vi "Clock Frequency generator hilbert.vi"(6 "Sweep Speed":dbl=20000.0 format="%#_13g", 8 "Error In":errorcluster, 9 "Acquisition speed (S/s)":i32=180000000, 10 "k-space signal in":u16[](array[numeric])=array[5000 elements], 11 "number of frequency updates":i32=4385) -> (0 "Error Out":errorcluster, 2 "frequency\nsteps":i32)   [LabVIEW 2014]
uses:
  <vilib>/Analysis/polynomials.llb/nth Derivative of Polynomial (DBL).vi
  <vilib>/Analysis/polynomials.llb/Scalar Polynomial Evaluation (DBL).vi
  <vilib>/Analysis/NI_AALPro.lvlib
panel:
  out "Frequency output 2":cluster{dbl[], dbl[]}[](graph)
  out "x*y":dbl[](array[numeric])
  out "Update time interval (ns)":dbl=10.0
  out "Frequency output":dbl[](graph)
  out "analytic phase":dbl[][](graph)
  in  "End of clock":i32=6300
  out "original signal":dbl[](graph)
  # "4385 updates is the maximum number for the clock of\nthe output card which updates every 11.4 ns"
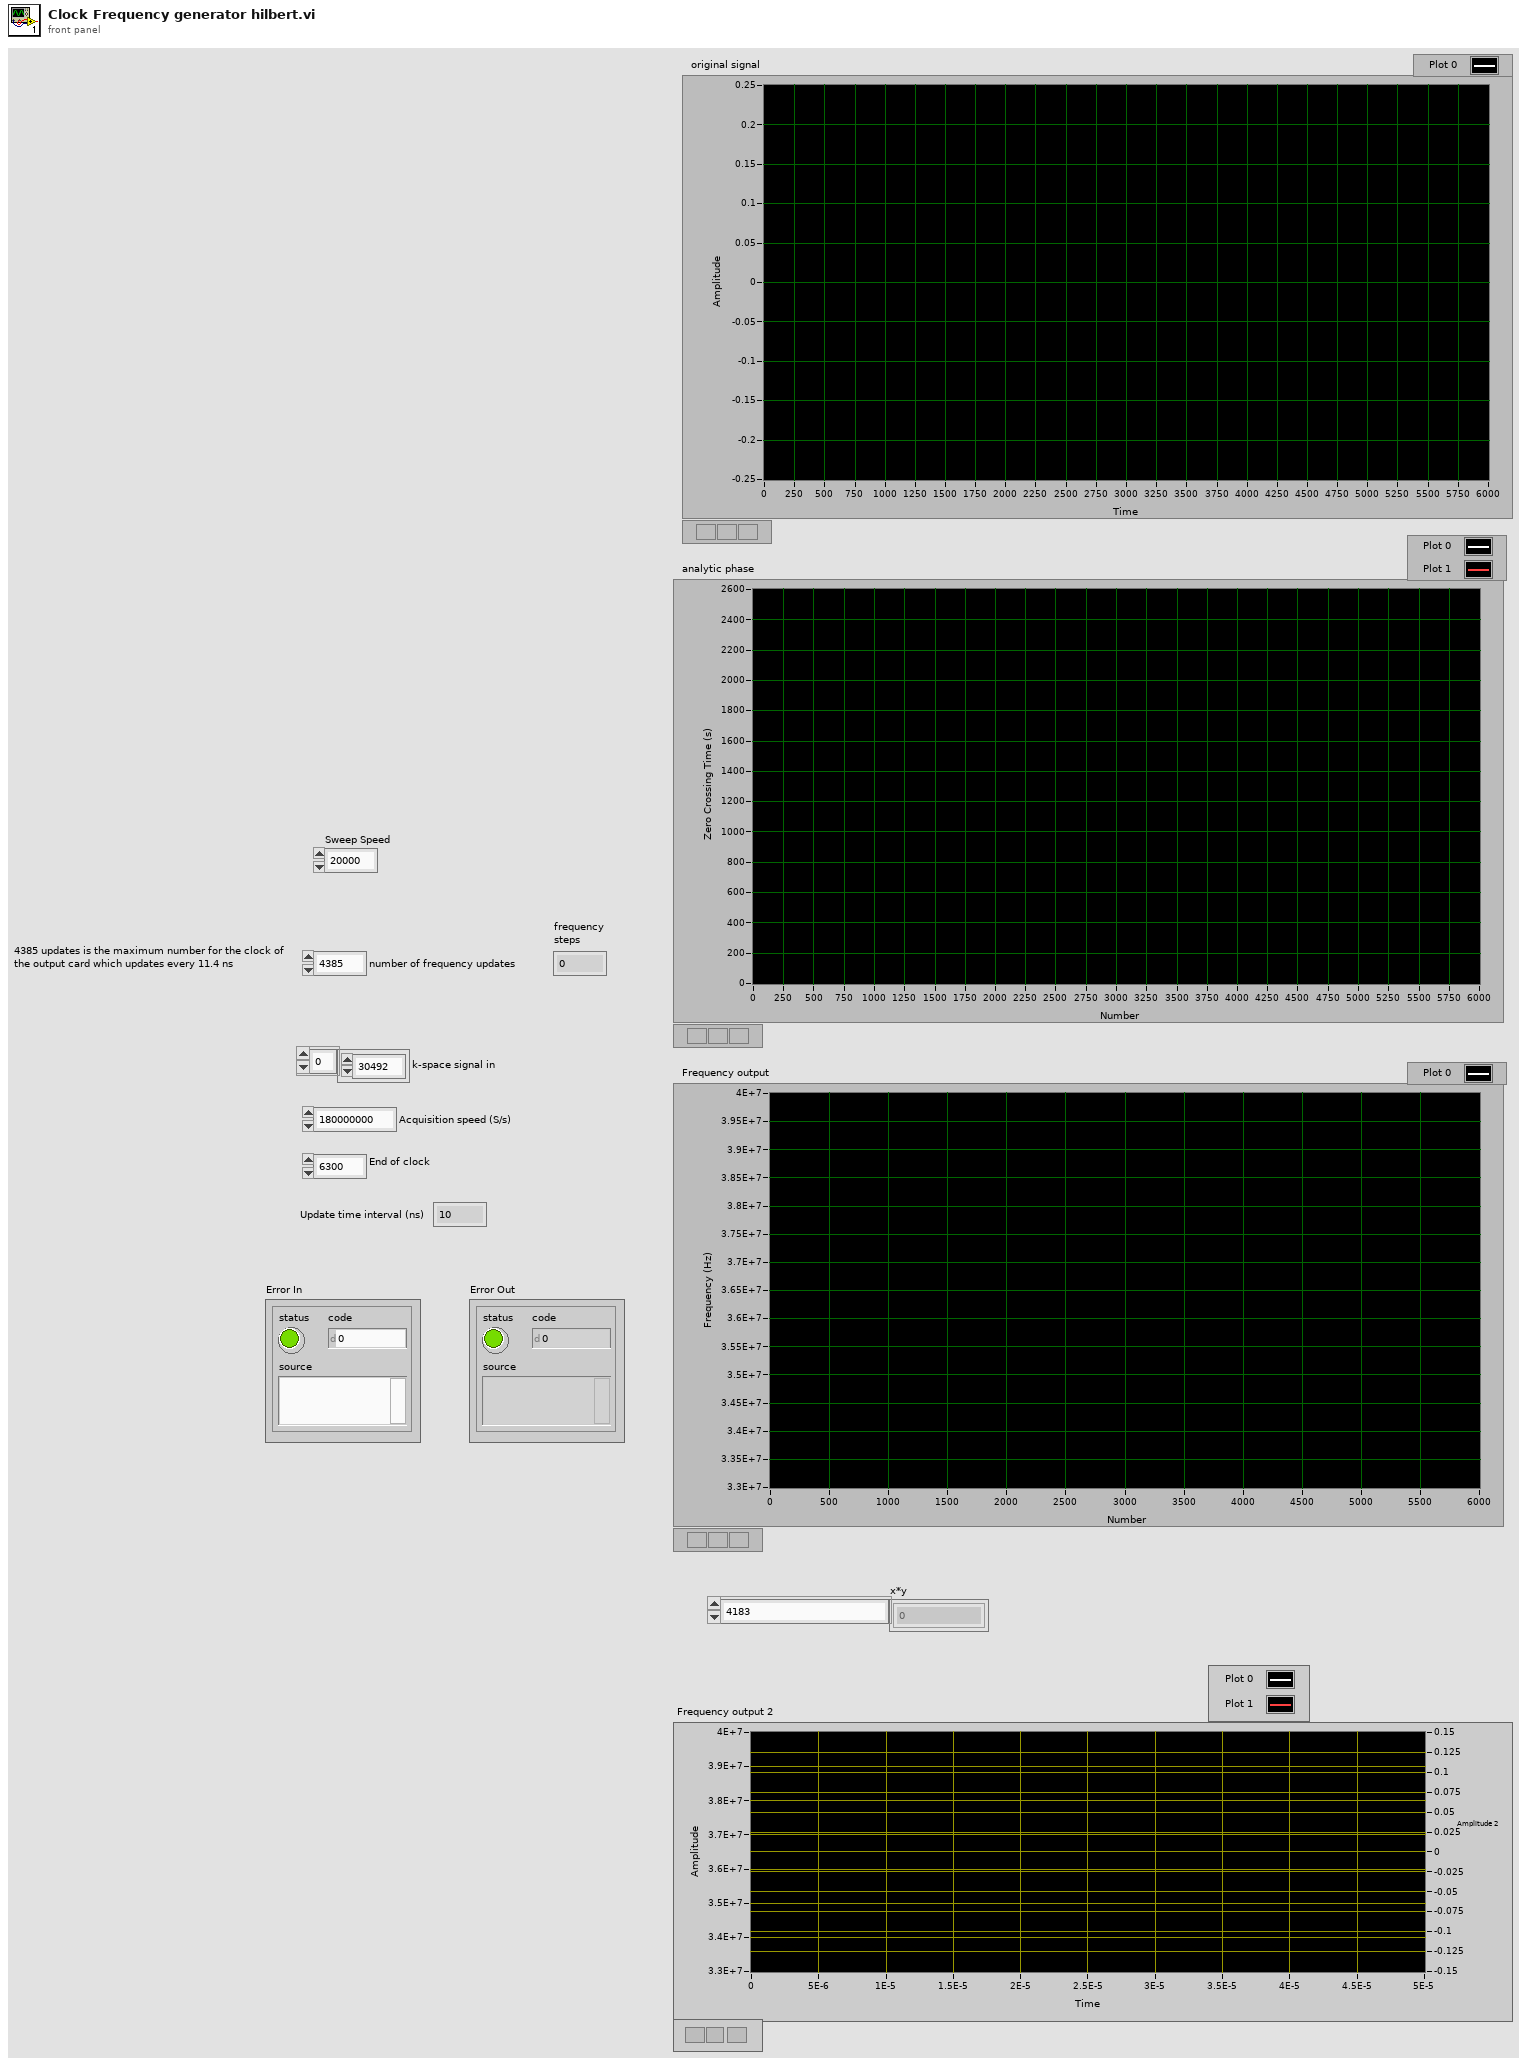
[diagram p1: front panel]
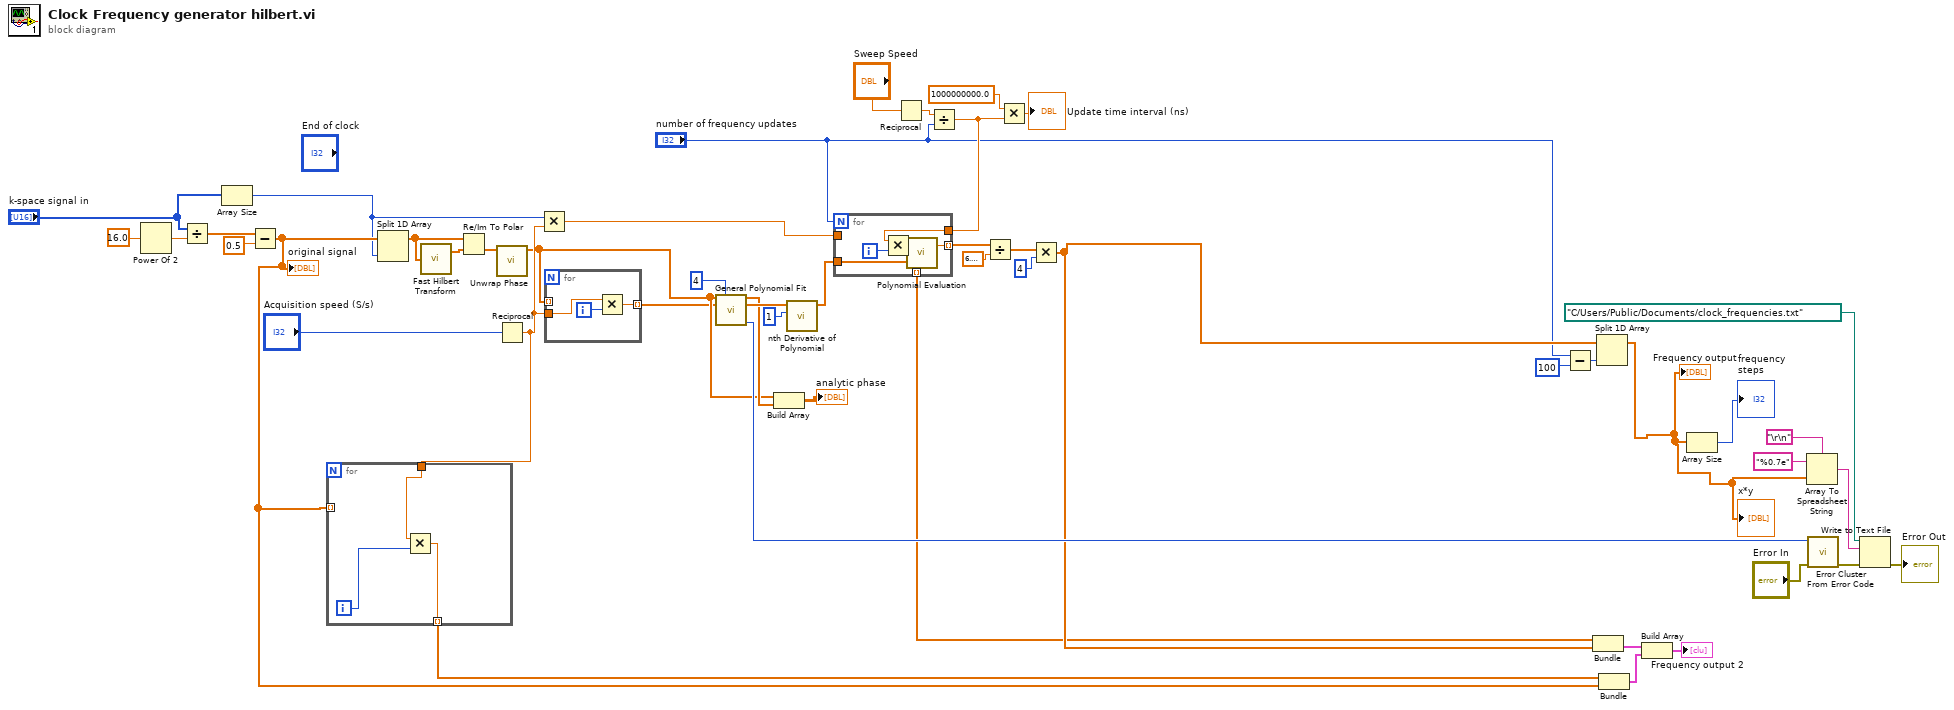
[diagram p0: block diagram]
diagram:
  n1 = Power Of 2(x=16.0) -> (2^x=w49:dbl)
  n2 = Divide(x="k-space signal in", y=w49) -> (x/y=w47:dbl[])
  n3 = Array Size(array="k-space signal in") -> (size(s)=w1:i32)
  n4 = Subtract(x=w47, y=0.5) -> (x-y=w12:dbl[])
  "original signal" <- w12
  n5 = Split 1D Array(array=w12, index=w1) -> (first subarray=w23:dbl[])  [unwired: 1 out]
  n6 = call <vilib>:"Fast Hilbert Transform.vi"("X"=w23) -> ("Hilbert{X}"=w26:dbl[])  [unwired: 1 out]
  n7 = Re/Im To Polar(2:w26, 3:w23) -> (0:w25:dbl[])  [unwired: 1 out]
  n8 = call <vilib>:"Unwrap Phase.vi"("Phase"=w25) -> ("Unwrapped Phase"=w8:dbl[])  [unwired: 9 in, 1 out]
  n9 = Reciprocal(x="Acquisition speed (S/s)") -> (1/x=w11:dbl)
  n10 = for {
    tunnel: w12 -> [_] mode=indexing
    tunnel: w11 -> [w52]
    tunnel: [w50] -> w9 mode=indexing
    i -> [w51]
    n11 = Multiply(x=w52, y=w51) -> (x*y=w50:dbl)
  }
  n12 = Multiply(x=w1, y=w11) -> (x*y=w22:dbl)
  n13 = for {
    tunnel: w8 -> [_] mode=indexing
    tunnel: [w54] -> w7 mode=indexing
    tunnel: w11 -> [w53]
    i -> [w55]
    n14 = Multiply(x=w53, y=w55) -> (x*y=w54:dbl)
  }
  n15 = call <vilib>:"General Polynomial Fit.vi"("Y"=w8, "polynomial order"=4, "X"=w7) -> ("Best Polynomial Fit"=w33:dbl[], "Polynomial Coefficients"=w36:dbl[], "error"=w30:i32)  [unwired: 9 in, 1 out]
  n16 = Build Array(w8, w33) -> (→"analytic phase":dbl[][])
  n17 = call-poly <vilib>:"nth Derivative of Polynomial.vi"("order"=1, "P(x)"=w36) -> ("Nth Derivative of P(x)"=w31:dbl[])  [unwired: 8 in, 1 out]
  n18 = Reciprocal(x="Sweep Speed") -> (1/x=w44:dbl)
  n19 = Divide(x=w44, y="number of frequency updates") -> (x/y=w17:dbl)
  n20 = for {
    N: "number of frequency updates" -> [_]
    tunnel: w31 -> [w59]
    tunnel: [w58] -> w19 mode=indexing
    tunnel: w22 -> [_]
    tunnel: [w57] -> w10 mode=indexing
    tunnel: w17 -> [w56]
    i -> [w60]
    n21 = Multiply(x=w56, y=w60) -> (x*y=w57:dbl)
    n22 = call-poly <vilib>:"Polynomial Evaluation.vi"("P(x)"=w59, "a"=w57) -> ("P(a)"=w58:dbl)  [unwired: 1 out]
  }
  n23 = Divide(x=w19, y=6.283185307179586) -> (x/y=w21:dbl[])
  n24 = Multiply(x=1000000000.0 ("y"), y=w17) -> (x*y=→"Update time interval (ns)":dbl)
  n25 = Multiply(x=w21, y=4 ("P(a)")) -> (x*y=w16:dbl[])
  n26 = Subtract(x="number of frequency updates", y=100) -> (x-y=w3:i32)
  n27 = Bundle(w10, w16) -> (w15:cluster{dbl[], dbl[]})  [unwired: 1 in]
  n28 = Split 1D Array(array=w16, index=w3) -> (first subarray=w6:dbl[])  [unwired: 1 out]
  "Frequency output" <- w6
  "x*y" <- w6
  n29 = Bundle(w9, w12) -> (w14:cluster{dbl[], dbl[]})  [unwired: 1 in]
  n30 = Build Array(w15, w14) -> (→"Frequency output 2":cluster{dbl[], dbl[]}[])
  n31 = Array Size(array=w6) -> (size(s)=→"frequency\nsteps":i32)
  n32 = Array To Spreadsheet String(delimiter (Tab)="\r\n", array=w6, 3:"%0.7e") -> (spreadsheet string=w41:string)
  n33 = call <vilib>:"Error Cluster From Error Code.vi"("error in (no error)"="Error In", "error code (0)"=w30) -> ("error out"=w28:errorcluster)  [unwired: 7 in]
  n34 = Write to Text File(file (use dialog)=path "C:/Users/Public/Documents/clock_frequencies.txt", text=w41, error in=w28) -> (error out=→"Error Out":errorcluster)  [unwired: 1 in, 2 out]
